vi "Schema Update.vi"(8 "error in (no error)":errorcluster, 10 "Schema":string, 11 "FE FF Frame in":refnum<class "FE FF Frame.lvclass">) -> (0 "error out":errorcluster, 3 "FE FF Frame out":refnum<class "FE FF Frame.lvclass">)   [LabVIEW 2023, in "Data Analysis.lvlib" / "FE FF Frame.lvlib" / "FE FF Frame.lvclass"]
uses:
  FE FF Frame.lvclass
  FE FF Frame.lvclass/FE FF Frame.ctl
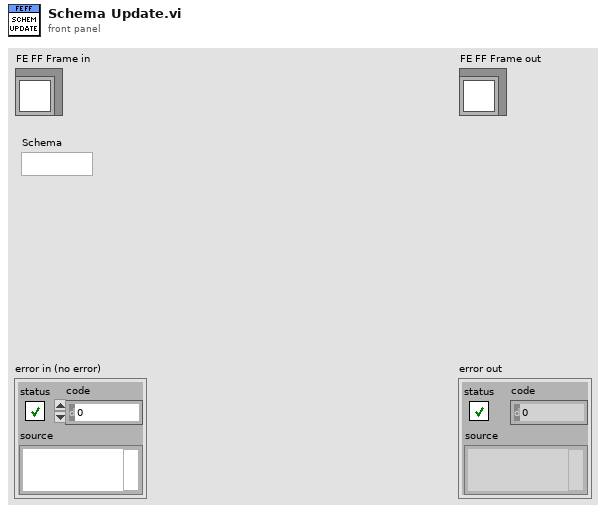
[diagram p1: front panel]
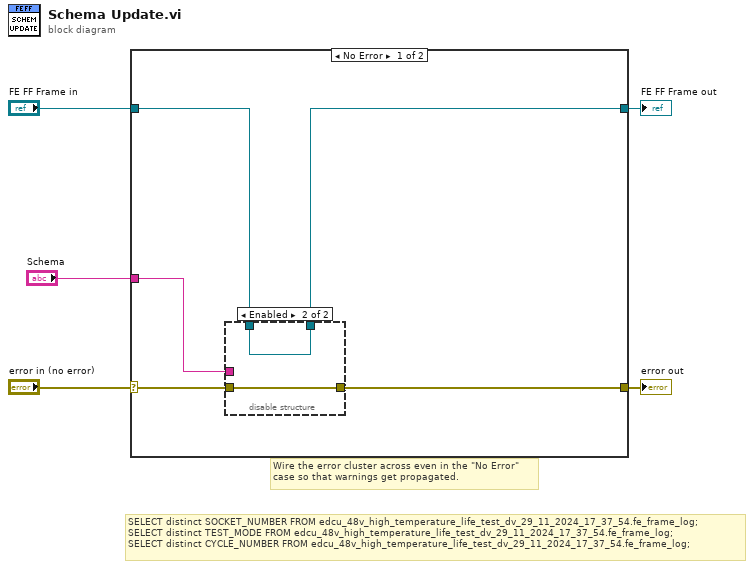
[diagram p0: block diagram]
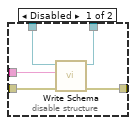
[diagram p2: hidden frame]
diagram:
  # "SELECT distinct SOCKET_NUMBER FROM edcu_48v_high_temperature_life_test_dv_29_11_2024_17_37_54.fe_frame_log;\nSELECT distinct TEST_MODE FROM edcu_48v_high_temperature_life_test_dv_29_11_2024_17_37_54.fe_frame_log;\nSELECT distinct CYCLE_NUMBER FROM edcu_48v_high_temperature_life_test_dv_29_11_2024_17_37_54.fe_frame_log;"
  # "Wire the error cluster across even in the \"No Error\"\ncase so that warnings get propagated."
  n1 = case shown="No Error" "error in (no error)" {
    selector: "error in (no error)" -> [w9 w19]
    tunnel: [w8 w19] -> w4
    tunnel: [w6 w18] -> w2
    tunnel: "FE FF Frame in" -> [w10 w18]
    tunnel: "Schema" -> [w7 _]
    frame No Error {
      n2 = disable-structure shown="Enabled" {
        disable-tunnel: w10 -> [w15 w17]
        disable-tunnel: w9 -> [w14 w16]
        disable-tunnel: [w13 w16] -> w8
        disable-tunnel: w7 -> [w12 _]
        disable-tunnel: [w11 w17] -> w6
        frame Disabled {
          n3 = call "Write Schema.vi"("error in (no error)"=w14, "Schema"=w12, "FE FF Frame in"=w15) -> ("error out"=w13:errorcluster, "FE FF Frame out"=w11:refnum<class "FE FF Frame.lvclass">)  [unwired: 7 in]
        }
        frame Enabled {
        }
      }
    }
    frame Error {
    }
  }
  "error out" <- w4
  "FE FF Frame out" <- w2
